vi "Generate Order Number.vi"(8 "error in (no error)":errorcluster, 11 "Cashier in":refnum<class "Cashier.lvclass">) -> (0 "error out":errorcluster, 2 "Order Number":u32, 3 "Cashier out":refnum<class "Cashier.lvclass">)   [LabVIEW 2023, in "Cashier.lvclass"]
doc: "Generates a random order number for simulation purposes."
uses:
  Cashier.lvclass
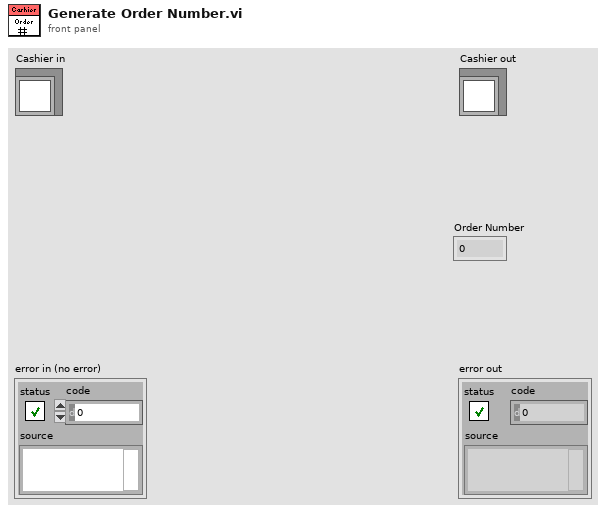
[diagram p1: front panel]
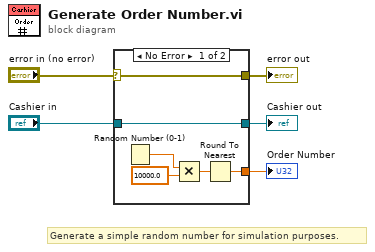
[diagram p0: block diagram]
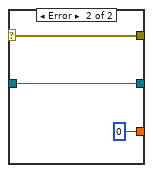
[diagram p2: hidden frame]
diagram:
  # "Generate a simple random number for simulation purposes."
  n1 = case shown="No Error" "error in (no error)" {
    selector: "error in (no error)" -> [w10 w14]
    tunnel: [w10 w14] -> w4
    tunnel: [w11 w13] -> w2
    tunnel: "Cashier in" -> [w11 w13]
    tunnel: [w6 u32 0 ("Order Number")] -> w1
    frame No Error {
      n2 = Random Number (0-1)() -> (number: 0 to 1=w9:dbl)
      n3 = Multiply(x=w9, y=10000.0) -> (x*y=w7:dbl)
      n4 = Round To Nearest(number=w7) -> (nearest integer value=w6:dbl)
    }
    frame Error {
    }
  }
  "error out" <- w4
  "Cashier out" <- w2
  "Order Number" <- w1
